vi "Find Build Spec.vi"(8 "error in (no error)":errorcluster, 10 "Build Spec Name":string, 11 "Target in":refnum<vi>) -> (0 "error out":errorcluster, 3 "Target":refnum<vi>)   [LabVIEW 2020, in "VolatusBuild.lvlib"]
uses:
  VolatusBuild.lvlib
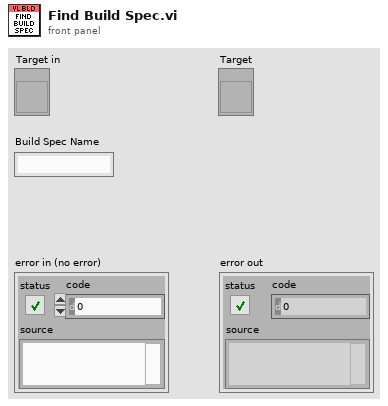
[diagram p1: front panel]
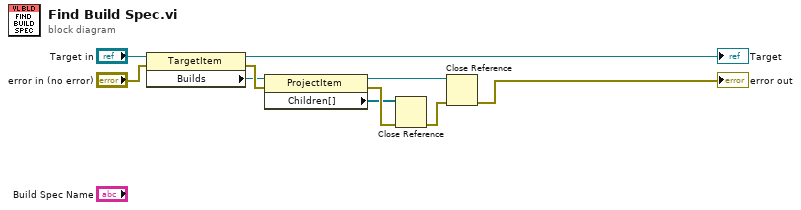
[diagram p0: block diagram]
diagram:
  n1 = property class="TargetItem"(reference="Target in", error in="error in (no error)") -> (reference out=→"Target":refnum<vi>, error out=w9:errorcluster, "Builds"=w5:refnum<vi>)
  n2 = property class="ProjectItem"(reference=w5, error in=w9) -> (reference out=w3:refnum<vi>, error out=w10:errorcluster, "Children[]"=w4:refnum<vi>[])
  n3 = Close Reference(reference=w4, error in (no error)=w10) -> (error out=w2:errorcluster)
  n4 = Close Reference(reference=w3, error in (no error)=w2) -> (error out=→"error out":errorcluster)
